vi "X-_parse_read.vi"(3 "Read":string, 5 "COMMAND":T1) -> (0 "String Reply":string, 2 "Numeric Reply":dbl format="%.2f")   [LabVIEW 2010]
uses:
  X-_commands.ctl
panel:
  out "force representation":i32
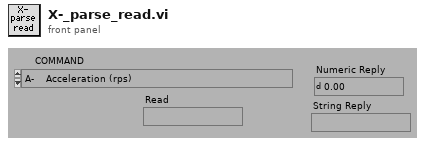
[diagram p1: front panel]
types:
  T1 = typedef "X-_commands.ctl" = enum16{"A-    Acceleration (rps)", "B-    Buffer Status", "C-    Continue", "CG-  Correction Gain", "CR-  Cariage Return", "D-    Distance (pulses)", "DB-  Dead Band (encoder steps)", "DW- Deadband Window (encoder steps)", "E-    Enable Communications", "ER-  Encoder Resolution (steps/rev)", "F-    Disable Communications", "FS-  Encoder Functions Report", "FSA- Incremental/Absolute (0/1)", "FSB- Motor/Encoder Step Mode (0/1)", "FSC- Enable/Disable Position Maint. (1/0)", "FSD- Stop/Continue on Stall (1/0)", "FSE- Activate o/p1 on Stall (1/0)", "FSF- Stop Motion on Trig3 (1/0)", "FSG- Activate o/p2 in Deadband (1/0)", "FSH- Enable Stall Detect (1/0)", "G- Go", "GH- Go Home and Zero (+/-V)", "^H- Delete ", "H- Direction Reverse/CCW/CW (0,1,2)", "IS- Input Status", "K- Kill", "L- Loop (n)", "LD- Limit DISABLE (0-none,1-CW,2-CCW,3-Both)", "LF- Line Feed", "MC- Mode Continuous", "MN- Mode Normal", "MPA- Motor Postion Absolute", "MPI- Motor Position Incremental", "MR- Motor Resolution (Drive Steps/rev)", "N- End of Loop", "O- Output (00,01,10,11)", "OS- Report Homing Setup", "OSA- NO/NC Limits (1/0)", "OSB- Back Up to Home/Edge? (0/1)", "OSC- NO/NC Home Switch (1/0)", "OSD- Enable Encoder Z for Home (0/1)", "OSH- Reference Edge for Home CW/CCW (0/1)", "PR- Report ABSOLUTE Position", "PS- Pause until Continue", "PX- Report Absolute ENCODER Position", "PZ- Zero Absolute Counter", "\"- Quote (17 ASCII +Space)", "Q- Enter/Exit Velocity Profiling (1/0)", "R- Request Indexer Status", "RA- Report Limit Switch Status", "RB- Report Loop, Pause, Shutdown, Trigger Status", "RC- Report Closed Loop Status", "RM- Velocity Streaming Rate Multiplier (000-FFF)", "RV- Report Revision Level", "S- Controlled Stop", "SN- Debounce (1-1000ms)", "SS- Report Software Switch Status", "SSA- Disable RS232 Echo (1/0)", "SSG- Clear/Save Command Buffer on Limit (0/1)", "SSH- Clear/Save Command Buffer on Stop (0/1)", "ST- Shutdown (1/0)", "SV- Servoing Setting (0,1,2,3)", "T- Time Delay (0.01-99999.99)", "TR- Wait for Trigger High/Low/Ignore (1/0/X)", "TS- Report Trigger Status", "U- Pause after Move Until Continue", "V- Velocity (0.01-50.00 revs/sec)", "W1- Report Relative Position <Signed Binary>", "W3- Report Relative Position <Hexadecimal>", "Y- Abort Loop at N", "Z-    Reset to Defaults", "#-    Disable/Set Soft Addresses (0/1-255)"}
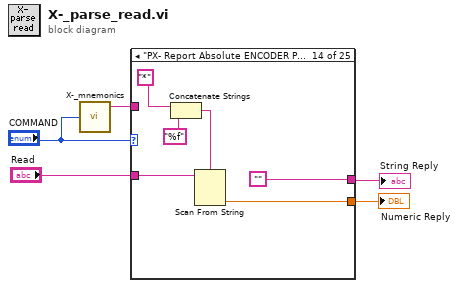
[diagram p0: block diagram]
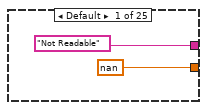
[diagram p2: hidden frame]
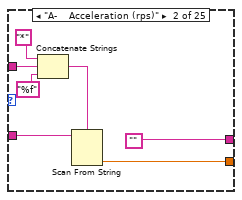
[diagram p3: hidden frame]
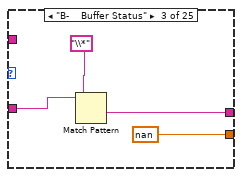
[diagram p4: hidden frame]
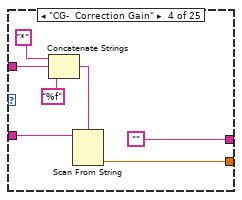
[diagram p5: hidden frame]
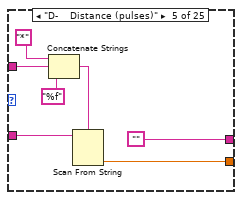
[diagram p6: hidden frame]
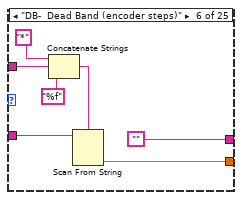
[diagram p7: hidden frame]
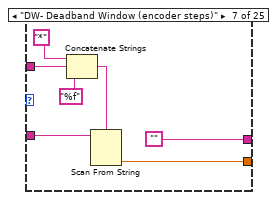
[diagram p8: hidden frame]
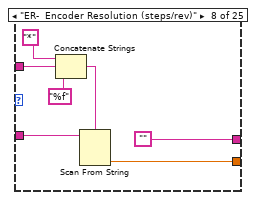
[diagram p9: hidden frame]
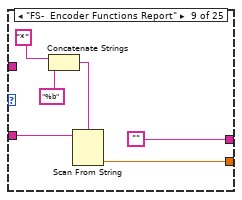
[diagram p10: hidden frame]
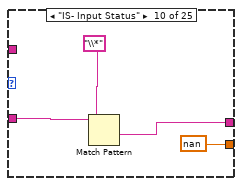
[diagram p11: hidden frame]
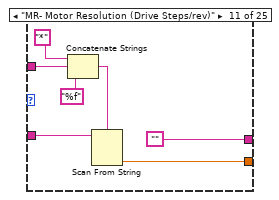
[diagram p12: hidden frame]
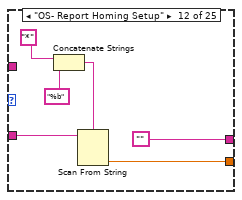
[diagram p13: hidden frame]
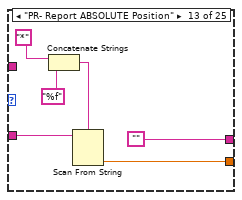
[diagram p14: hidden frame]
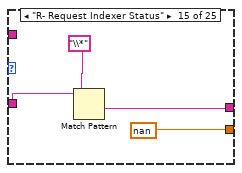
[diagram p15: hidden frame]
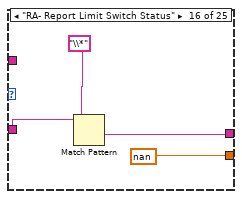
[diagram p16: hidden frame]
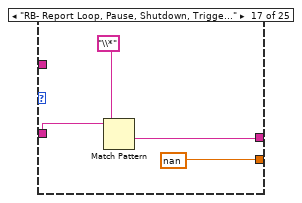
[diagram p17: hidden frame]
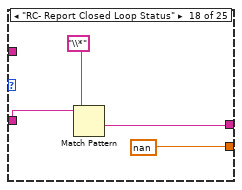
[diagram p18: hidden frame]
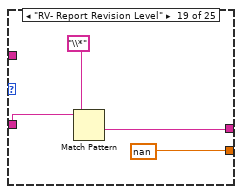
[diagram p19: hidden frame]
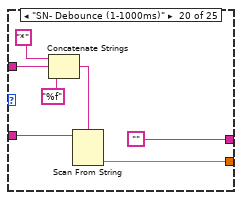
[diagram p20: hidden frame]
diagram:
  n1 = call "X-_mnemonics.vi"("COMMAND"="COMMAND") -> ("Mnemonic"=w5:string)  [unwired: 2 out]
  n2 = case shown="\"PX- Report Absolute ENCODER Position\"" "COMMAND" {
    tunnel: "Read" -> [_ w14 w18 w24 w31 w38 w45 w52 w58 w62 w69 w71 w81 w88 w91 w95 w99 w103 w107 w114 w116 w126 w133 w135 w144]
    tunnel: w5 -> [_ w10 _ w20 w27 w34 w41 w48 _ _ w65 _ _ _ _ _ _ _ _ w110 _ _ w129 _ _]
    tunnel: ["Not Readable" "" w17 "" "" "" "" "" "" w61 "" "" "" "" w90 w94 w98 w102 w106 "" "" "" "" "" ""] -> w3
    tunnel: [nan w9 nan w23 w30 w37 w44 w51 w57 nan w68 w73 w80 w87 nan nan nan nan nan w113 w117 w125 w132 w136 w140] -> w4
    frame Default {
    }
    frame "A-    Acceleration (rps)" {
      n3 = Concatenate Strings("*", w10, "%f") -> (w12:string)
      n4 = Scan From String(format string=w12, input string=w14) -> (output 1=w9:dbl)  [unwired: 2 in, 4 out]
    }
    frame "B-    Buffer Status" {
      n5 = Match Pattern(string=w18, regular expression="\\*") -> (after substring=w17:string)  [unwired: 4 out]
    }
    frame "CG-  Correction Gain" {
      n6 = Concatenate Strings("*", w20, "%f") -> (w21:string)
      n7 = Scan From String(format string=w21, input string=w24) -> (output 1=w23:dbl)  [unwired: 2 in, 4 out]
    }
    frame "D-    Distance (pulses)" {
      n8 = Concatenate Strings("*", w27, "%f") -> (w28:string)
      n9 = Scan From String(format string=w28, input string=w31) -> (output 1=w30:dbl)  [unwired: 2 in, 4 out]
    }
    frame "DB-  Dead Band (encoder steps)" {
      n10 = Concatenate Strings("*", w34, "%f") -> (w35:string)
      n11 = Scan From String(format string=w35, input string=w38) -> (output 1=w37:dbl)  [unwired: 2 in, 4 out]
    }
    frame "DW- Deadband Window (encoder steps)" {
      n12 = Concatenate Strings("*", w41, "%f") -> (w42:string)
      n13 = Scan From String(format string=w42, input string=w45) -> (output 1=w44:dbl)  [unwired: 2 in, 4 out]
    }
    frame "ER-  Encoder Resolution (steps/rev)" {
      n14 = Concatenate Strings("*", w48, "%f") -> (w49:string)
      n15 = Scan From String(format string=w49, input string=w52) -> (output 1=w51:dbl)  [unwired: 2 in, 4 out]
    }
    frame "FS-  Encoder Functions Report" {
      n16 = Concatenate Strings("*", "%b") -> (w56:string)
      n17 = Scan From String(format string=w56, input string=w58) -> (output 1=w57:dbl)  [unwired: 2 in, 4 out]
    }
    frame "IS- Input Status" {
      n18 = Match Pattern(string=w62, regular expression="\\*") -> (after substring=w61:string)  [unwired: 4 out]
    }
    frame "MR- Motor Resolution (Drive Steps/rev)" {
      n19 = Concatenate Strings("*", w65, "%f") -> (w66:string)
      n20 = Scan From String(format string=w66, input string=w69) -> (output 1=w68:dbl)  [unwired: 2 in, 4 out]
    }
    frame "OS- Report Homing Setup" {
      n21 = Concatenate Strings("*", "%b") -> (w75:string)
      n22 = Scan From String(format string=w75, input string=w71) -> (output 1=w73:dbl)  [unwired: 2 in, 4 out]
    }
    frame "PR- Report ABSOLUTE Position" {
      n23 = Concatenate Strings("*", "%f") -> (w79:string)
      n24 = Scan From String(format string=w79, input string=w81) -> (output 1=w80:dbl)  [unwired: 2 in, 4 out]
    }
    frame "PX- Report Absolute ENCODER Position" {
      n25 = Concatenate Strings("*", "%f") -> (w85:string)
      n26 = Scan From String(format string=w85, input string=w88) -> (output 1=w87:dbl)  [unwired: 2 in, 4 out]
    }
    frame "R- Request Indexer Status" {
      n27 = Match Pattern(string=w91, regular expression="\\*") -> (after substring=w90:string)  [unwired: 4 out]
    }
    frame "RA- Report Limit Switch Status" {
      n28 = Match Pattern(string=w95, regular expression="\\*") -> (after substring=w94:string)  [unwired: 4 out]
    }
    frame "RB- Report Loop, Pause, Shutdown, Trigger Status" {
      n29 = Match Pattern(string=w99, regular expression="\\*") -> (after substring=w98:string)  [unwired: 4 out]
    }
    frame "RC- Report Closed Loop Status" {
      n30 = Match Pattern(string=w103, regular expression="\\*") -> (after substring=w102:string)  [unwired: 4 out]
    }
    frame "RV- Report Revision Level" {
      n31 = Match Pattern(string=w107, regular expression="\\*") -> (after substring=w106:string)  [unwired: 4 out]
    }
    frame "SN- Debounce (1-1000ms)" {
      n32 = Concatenate Strings("*", w110, "%f") -> (w111:string)
      n33 = Scan From String(format string=w111, input string=w114) -> (output 1=w113:dbl)  [unwired: 2 in, 4 out]
    }
    frame "SS- Report Software Switch Status" {
      n34 = Concatenate Strings("*", "%b") -> (w120:string)
      n35 = Scan From String(format string=w120, input string=w116) -> (output 1=w117:dbl)  [unwired: 2 in, 4 out]
    }
    frame "TS- Report Trigger Status" {
      n36 = Concatenate Strings("*", "%b3") -> (w124:string)
      n37 = Scan From String(format string=w124, input string=w126) -> (output 1=w125:dbl)  [unwired: 2 in, 4 out]
    }
    frame "V- Velocity (0.01-50.00 revs/sec)" {
      n38 = Concatenate Strings("*", w129, "%f") -> (w130:string)
      n39 = Scan From String(format string=w130, input string=w133) -> (output 1=w132:dbl)  [unwired: 2 in, 4 out]
    }
    frame "W1- Report Relative Position <Signed Binary>" {
      n40 = String To Byte Array(string=w135) -> (unsigned byte array=w138:u8[])
      n41 = Type Cast(type=0, x=w138) -> (*(type *) &x=w136:i32)
    }
    frame "W3- Report Relative Position <Hexadecimal>" {
      n42 = Concatenate Strings("*", "%x8") -> (w146:string)
      n43 = Scan From String(format string=w146, input string=w144) -> (output 1=w141:i32)  [unwired: 2 in, 4 out]
      "force representation" <- w141
      n44 = To Double Precision Float(number=w141) -> (double precision float=w140:dbl)
    }
  }
  "Numeric Reply" <- w4
  "String Reply" <- w3
